vi "Config PGA.vi"(1 "PGA":T1(ring), 2 "Orig Config":u8[](array[numeric])) -> (0 "New Config":u8[](array[numeric]))   [LabVIEW 2021]
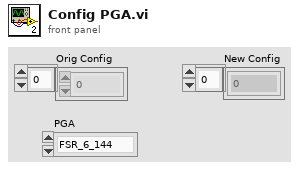
[diagram p1: front panel]
types:
  T1 = enum16{"FSR_6_144", "FSR_4_096", "FSR_2_048", "FSR_1_024", "FSR_0_512", "FSR_0_256"}
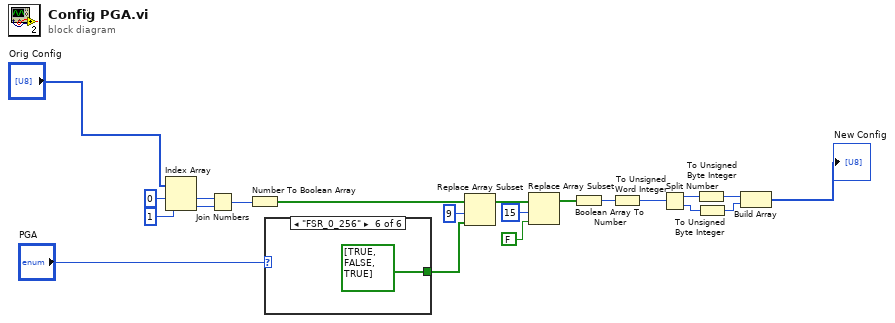
[diagram p0: block diagram]
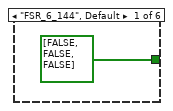
[diagram p2: hidden frame]
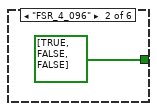
[diagram p3: hidden frame]
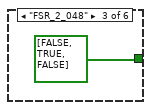
[diagram p4: hidden frame]
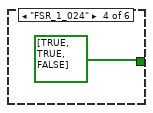
[diagram p5: hidden frame]
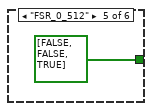
[diagram p6: hidden frame]
diagram:
  n1 = Index Array(array="Orig Config", index #1=0 ("index"), index #2=1 ("index")) -> (element #1=w4:u8, element #2=w5:u8)
  n2 = Join Numbers(hi=w4, lo=w5) -> ((hi.lo)=w6:u16)
  n3 = Number To Boolean Array(number=w6) -> (Boolean array=w7:bool[])
  n4 = case shown="\"FSR_0_256\"" "PGA" {
    tunnel: [bool[] [FALSE, FALSE, FALSE] bool[] [TRUE, FALSE, FALSE] bool[] [FALSE, TRUE, FALSE] bool[] [TRUE, TRUE, FALSE] bool[] [FALSE, FALSE, TRUE] bool[] [TRUE, FALSE, TRUE]] -> w9
    frame "FSR_6_144", Default {
    }
    frame "FSR_4_096" {
    }
    frame "FSR_2_048" {
    }
    frame "FSR_1_024" {
    }
    frame "FSR_0_512" {
    }
    frame "FSR_0_256" {
    }
  }
  n5 = Replace Array Subset(array=w7, new element=w9, index=9) -> (w17:bool[])
  n6 = Replace Array Subset(array=w17, new element=FALSE ("new element/subarray"), index=15) -> (w20:bool[])
  n7 = Boolean Array To Number(Boolean array=w20) -> (number=w14:u32)
  n8 = To Unsigned Word Integer(number=w14) -> (unsigned 16bit integer=w15:u16)
  n9 = Split Number(x=w15) -> (hi(x)=w10:u8, lo(x)=w12:u8)
  n10 = To Unsigned Byte Integer(number=w10) -> (unsigned 8bit integer=w11:u8)
  n11 = To Unsigned Byte Integer(number=w12) -> (unsigned 8bit integer=w13:u8)
  n12 = Build Array(w11, w13) -> (→"New Config":u8[])
